vi "Embed Logo.vi"(10 "LogoPath":path, 11 "MissionLogo in":refnum<vi>) -> (3 "MissionLogo out":refnum<vi>)   [LabVIEW 2019, in "Test Selector.lvlib" / "Test Selector.lvclass"]
uses:
  Test Selector.lvclass
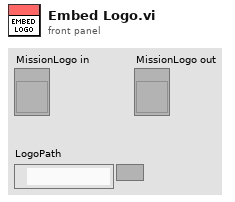
[diagram p1: front panel]
types:
  T1 = typedef "imagedata.ctl" = cluster{"image type":i32, "image depth":i32, "image":u8[], "mask":u8[], "colors":u32[], "Rectangle":cluster{"left":i16, "top":i16, "right":i16, "bottom":i16}}
  T2 = typedef "LVBoundsTypeDef.ctl" = cluster{"Width":u32, "Height":u32}
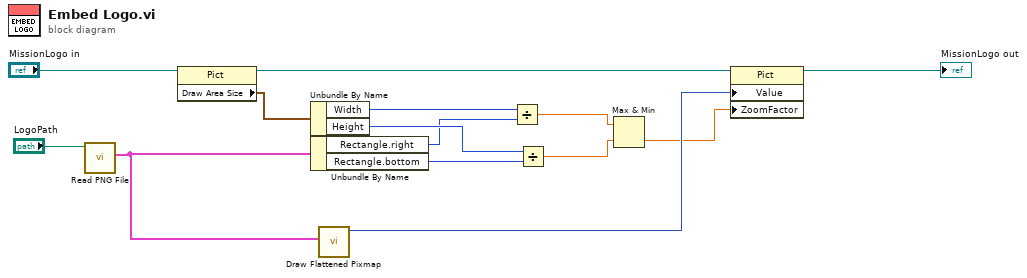
[diagram p0: block diagram]
diagram:
  n1 = call <vilib>:"Read PNG File.vi"("path to PNG file"="LogoPath") -> ("image data"=w1:T1)  [unwired: 8 in, 2 out]
  n2 = property class="Pict"(reference="MissionLogo in") -> (reference out=w6:refnum<vi>, "Draw Area Size"=w9:T2)  [unwired: 1 in, 1 out]
  n3 = Unbundle By Name(w9) -> ("Width"=w12:u32, "Height"=w13:u32)
  n4 = Unbundle By Name(w1) -> ("Rectangle.right"=w7:i16, "Rectangle.bottom"=w8:i16)
  n5 = call <vilib>:"Draw Flattened Pixmap.vi"("image data"=w1) -> ("new picture"=w4:picture)  [unwired: 8 in]
  n6 = Divide(x=w12, y=w7) -> (x/y=w10:dbl)
  n7 = Divide(x=w13, y=w8) -> (x/y=w11:dbl)
  n8 = Max & Min(x=w10, y=w11) -> (min(x,y)=w3:dbl)  [unwired: 1 out]
  n9 = property class="Pict"(reference=w6, "Value"=w4, "ZoomFactor"=w3) -> (reference out=→"MissionLogo out":refnum<vi>)  [unwired: 1 in, 1 out]
